vi "NII32ToFunctionEnum.vi"(11 "NI Function in":i32) -> (3 "Function out":T1)   [LabVIEW 2020, in "NI DMM Driver.lvlib" / "DMM.NI.lvclass"]
doc: "Convert the function I32 read from the NI DMM to the DMM Driver enum."
uses:
  DMM.NI.lvclass
  PPL/HDH.Driver.DMM.lvlibp/Controls/Ctl_Function.ctl
  PPL/HDH.Driver.DMM.lvlibp
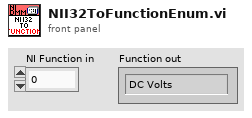
[diagram p1: front panel]
types:
  T1 = typedef "HDH.Driver.DMM.lvlibp/Ctl_Function.ctl" = enum8{"DC Volts", "AC Volts", "DC Current", "AC Current", "2-wire Resistance", "4-wire Resistance", "Diode", "Frequency", "Period", "AC Volts DC Coupled", "Capacitance", "Inductance", "Temperature"}
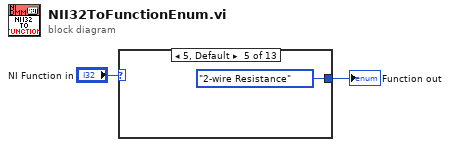
[diagram p0: block diagram]
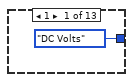
[diagram p2: hidden frame]
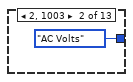
[diagram p3: hidden frame]
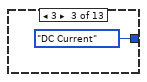
[diagram p4: hidden frame]
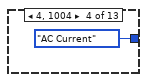
[diagram p5: hidden frame]
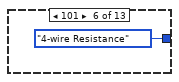
[diagram p6: hidden frame]
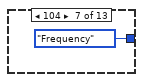
[diagram p7: hidden frame]
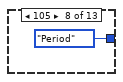
[diagram p8: hidden frame]
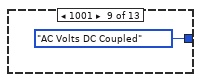
[diagram p9: hidden frame]
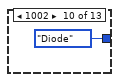
[diagram p10: hidden frame]
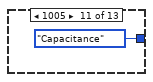
[diagram p11: hidden frame]
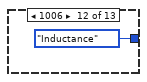
[diagram p12: hidden frame]
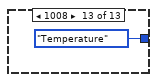
[diagram p13: hidden frame]
diagram:
  n1 = case shown="5, Default" "NI Function in" {
    tunnel: [Ctl_Function."DC Volts" ("Function") Ctl_Function."AC Volts" ("Function") Ctl_Function."DC Current" ("Function") Ctl_Function."AC Current" ("Function") Ctl_Function."2-wire Resistance" ("Function") Ctl_Function."4-wire Resistance" ("Function") Ctl_Function."Frequency" ("Function") Ctl_Function."Period" ("Function") Ctl_Function."AC Volts DC Coupled" ("Function") Ctl_Function."Diode" ("Function") Ctl_Function."Capacitance" ("Function") Ctl_Function."Inductance" ("Function") Ctl_Function."Temperature" ("Function")] -> w2
    frame 1 {
    }
    frame 2, 1003 {
    }
    frame 3 {
    }
    frame 4, 1004 {
    }
    frame 5, Default {
    }
    frame 101 {
    }
    frame 104 {
    }
    frame 105 {
    }
    frame 1001 {
    }
    frame 1002 {
    }
    frame 1005 {
    }
    frame 1006 {
    }
    frame 1008 {
    }
  }
  "Function out" <- w2
